vi "3D Point Cloud Display LV12 - NI Verified.vi"() -> ()   [LabVIEW 2012]
uses:
  <vilib>/Utility/miscctls.llb/LVRGBAColorTypeDef.ctl
  <vilib>/Utility/miscctls.llb/LV3DPointTypeDef.ctl
  <vilib>/picture/3D Picture Control/NI_3D Picture Control.lvlib
panel:
  in  "file path (dialog if empty)":path
  in  "From File?":bool
  in  "Camera Controller:":T1(ring)=enum."Spherical"
  in  "stop":bool
  out "3D Picture":refnum<vi>(3d-picture)
  # "Overview:  Code that shows how to load a 3D point cloud data into a 3D picture control in LabVIEW.\nRequirements: LabVIEW 2012 or compatible\nInstructions:\n1. Select if you would like to load from file or generate a random object.\n2. Run the VI.\n3. Use the Camera Controller to adjust the way the mouse moves the 3D object."
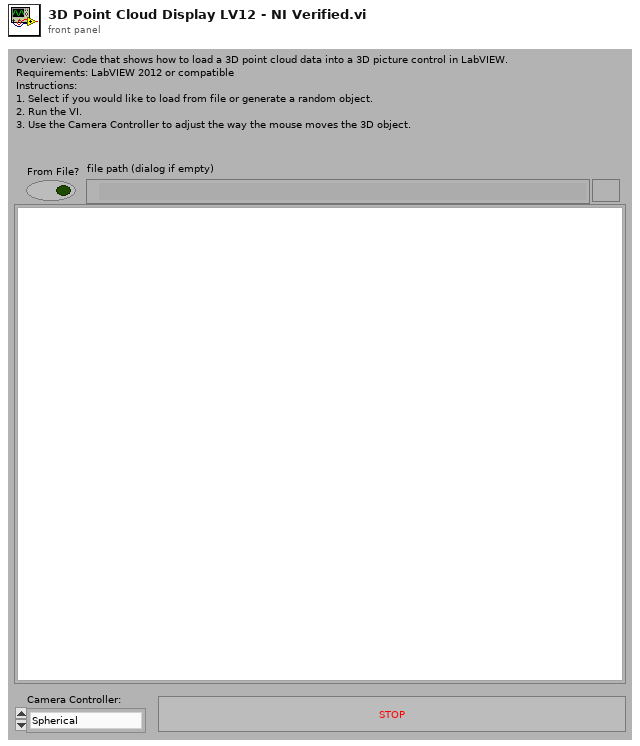
[diagram p1: front panel]
types:
  T1 = enum16{"None", "Spherical", "Flying", "Oriented"}
  T2 = typedef "LVRGBAColorTypeDef.ctl" = cluster{"Red":sgl, "Green":sgl, "Blue":sgl, "Alpha":sgl}
  T3 = enum16{"Overall", "Per Primitive", "Per Vertex", "Binding Off"}
  T4 = enum16{"Points", "Lines", "Line Strip", "Line Loop", "Triangles", "Triangle Strip", "Triangle Fan", "Quads", "Quad Strip", "Polygon"}
  T5 = typedef "LV3DPointTypeDef.ctl" = cluster{"X":sgl, "Y":sgl, "Z":sgl}
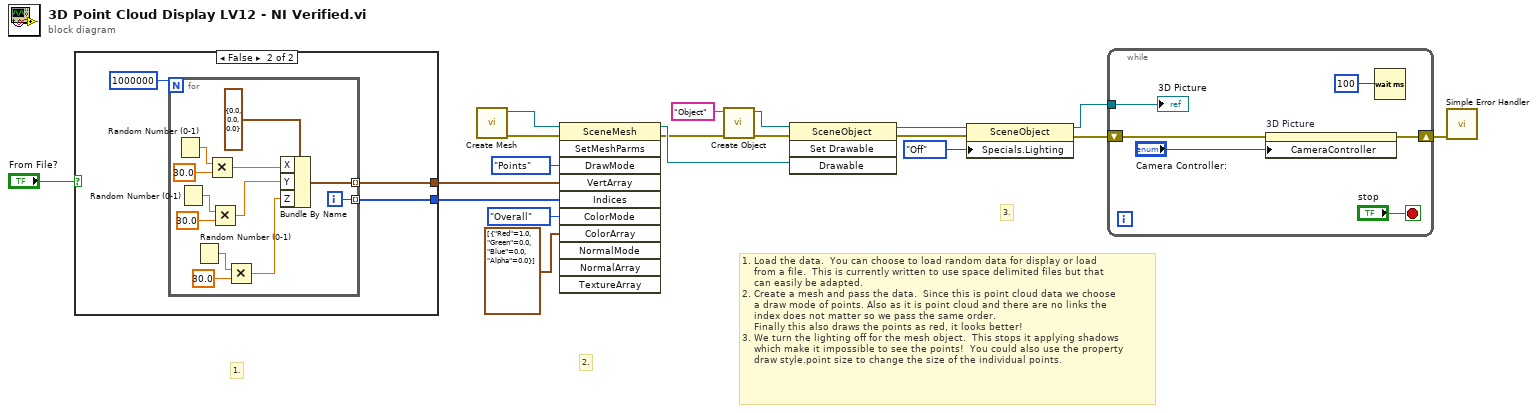
[diagram p0: block diagram]
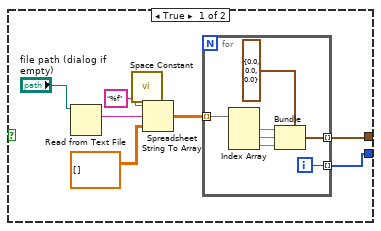
[diagram p2: hidden frame]
diagram:
  # "1. Load the data.  You can choose to load random data for display or load \n    from a file.  This is currently written to use space delimited files but that\n    can easily be adapted.\n2. Create a mesh and pass the data.  Since this is point cloud data we choose\n    a draw mode of points. Also as it is point cloud and there are no links the \n    index does not matter so we pass the same order.\n    Finally this also draws the points as red, it looks better!\n3. We turn the lighting off for the mesh object.  This stops it applying shadows\n    which make it impossible to see the points!  You could also use the property\n    draw style.point size to change the size of the individual points."
  # "3."
  # "2."
  # "1."
  n1 = case shown="False" "From File?" {
    tunnel: [w21 w36] -> w17
    tunnel: [w20 w35] -> w7
    frame True {
      n2 = Read from Text File(file (use dialog)="file path (dialog if empty)") -> (text=w26:string)  [unwired: 3 in, 3 out]
      n3 = call <vilib>:"Space Constant.vi"() -> ("String"=w25:string)
      n4 = Spreadsheet String To Array(delimiter (Tab)=w25, format string="%f", spreadsheet string=w26, array type (2D Dbl)=sgl[][] []) -> (array=w23:sgl[][])
      n5 = for {
        tunnel: w23 -> [w34] mode=indexing
        tunnel: [w29] -> w21 mode=indexing
        tunnel: [w28] -> w20 mode=indexing
        i -> [w28]
        n6 = Index Array(array=w34) -> (element #1=w32:sgl, element #2=w31:sgl, element #3=w30:sgl)  [unwired: 3 in]
        n7 = Bundle(cluster=T5 {"X"=0.0, "Y"=0.0, "Z"=0.0} ("3D Point"), "X"=w32, "Y"=w31, "Z"=w30) -> (w29:T5)
      }
    }
    frame False {
      n8 = for {
        N: 1000000 -> [_]
        tunnel: [w39] -> w36 mode=indexing
        tunnel: [w38] -> w35 mode=indexing
        i -> [w38]
        n9 = Random Number (0-1)() -> (number: 0 to 1=w47:dbl)
        n10 = Random Number (0-1)() -> (number: 0 to 1=w46:dbl)
        n11 = Random Number (0-1)() -> (number: 0 to 1=w43:dbl)
        n12 = Multiply(x=w47, y=30.0) -> (x*y=w42:dbl)
        n13 = Multiply(x=w46, y=30.0) -> (x*y=w41:dbl)
        n14 = Multiply(x=w43, y=30.0) -> (x*y=w40:dbl)
        n15 = Bundle By Name(cluster=T5 {"X"=0.0, "Y"=0.0, "Z"=0.0} ("3D Point"), "X"=w42, "Y"=w41, "Z"=w40) -> (w39:T5)
      }
    }
  }
  n16 = call <vilib>:"Create Mesh.vi"() -> ("error out"=w6:errorcluster, "New Mesh Refnum"=w15:refnum<vi>)  [unwired: 10 in]
  n17 = invoke class="SceneMesh" method="SetMeshParms"(reference=w15, error in=w6, "DrawMode"=T4."Points" ("Draw Mode"), "VertArray"=w17, "Indices"=w7, "ColorMode"=T3."Overall" ("Color Binding Mode"), "ColorArray"=T2[] [{"Red"=1.0, "Green"=0.0, "Blue"=0.0, "Alpha"=0.0}] ("Color Array")) -> (reference out=w11:refnum<vi>, error out=w3:errorcluster)  [unwired: 4 in, 9 out]
  n18 = call <vilib>:"Create Object.vi"("error in (no error)"=w3, "Name"="Object") -> ("error out"=w2:errorcluster, "Scene:New Object"=w18:refnum<vi>)  [unwired: 8 in]
  n19 = invoke class="SceneObject" method="Set Drawable"(reference=w18, error in=w2, "Drawable"=w11) -> (reference out=w10:refnum<vi>, error out=w5:errorcluster)  [unwired: 1 in, 2 out]
  n20 = property class="SceneObject"(reference=w10, error in=w5, "Specials.Lighting"=enum16{"Inherit Value", "Off", "On"}."Off" ("Specials:Lighting")) -> (reference out=w9:refnum<vi>, error out=w4:errorcluster)
  n21 = while {
    tunnel: w9 -> [w55]
    shift-right: [w50] -> w1
    shift-left: w4 -> [w51]
    stop <- "stop" stop-if-true
    n22 = property on="3D Picture" class="SceneGraphDisp (strict)"(error in=w51, "CameraController"="Camera Controller:") -> (error out=w50:errorcluster)  [unwired: 1 in, 1 out]
    n23 = Wait (ms)(milliseconds to wait=u32 100 ("millisecond multiple")) -> ()  [unwired: 1 out]
    "3D Picture" <- w55
  }
  n24 = call <vilib>:"Simple Error Handler.vi"("error in (no error)"=w1) -> ()  [unwired: 4 in, 5 out]
